vi "FetchLast_N_Records(SubVI).vi"(7 "# of Records":i32=10, 11 "Data In in":string[][](array[string])) -> (3 "Data In out":string[][](array[string]))   [LabVIEW 2018, in "DS_Lib.lvlib" / "SRReportParser.lvlib"]
uses:
  SRReportParser.lvlib
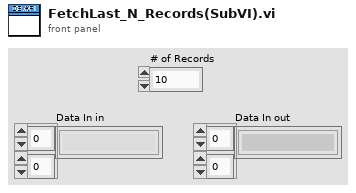
[diagram p1: front panel]
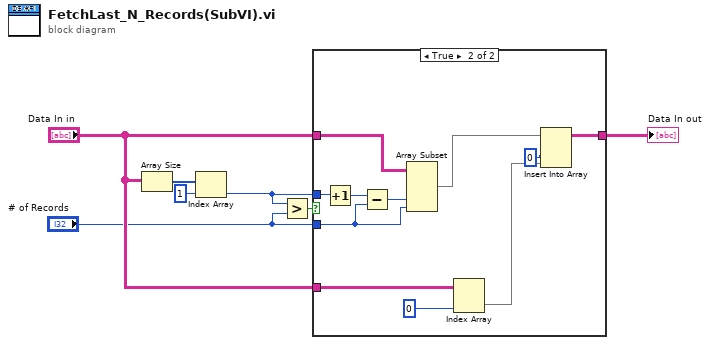
[diagram p0: block diagram]
diagram:
  n1 = Array Size(array="Data In in") -> (size(s)=w3:i32[])
  n2 = Index Array(array=w3, index=1) -> (element=w6:i32)
  n3 = Greater?(x=w6, y="# of Records") -> (0:w4:bool)
  n4 = case shown="True" w4 {
    tunnel: "Data In in" -> [w8 w18]
    tunnel: [w8 w13] -> w5
    tunnel: w6 -> [_ w10]
    tunnel: "# of Records" -> [_ w12]
    tunnel: "Data In in" -> [_ w11]
    frame False {
    }
    frame True {
      n5 = Increment(x=w10) -> (x+1=w9:i32)
      n6 = Subtract(x=w9, y=w12) -> (x-y=w19:i32)
      n7 = Array Subset(array=w18, index (col)=w19, length (col)=w12) -> (w16:string[][])  [unwired: 2 in]
      n8 = Index Array(array=w11, index (col)=0 ("disabled index (col)")) -> (element=w14:string[])  [unwired: 1 in]
      n9 = Insert Into Array(array=w16, index (col)=0 ("disabled index (col)"), new element=w14) -> (w13:string[][])  [unwired: 1 in]
    }
  }
  "Data In out" <- w5
